vi "ADC.vi"() -> ()   [LabVIEW 2012]
panel:
  out "Current Guess 2":dbl
  out "ADC Output":dbl
  out "Current Guess":dbl
  in  "Slow Conversion?":bool
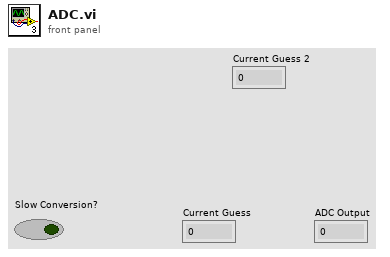
[diagram p1: front panel]
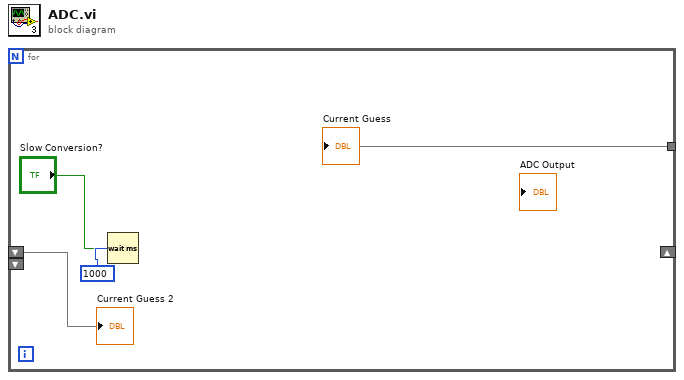
[diagram p0: block diagram]
diagram:
  n1 = for {
    shift-right: _ -> [_]
    shift-left: _ -> [w2]
    shift-left: _ -> [_]
    tunnel: _ -> [w1]
    n2 = Wait (ms)(milliseconds to wait=u32 1000 ("millisecond timer value"), millisecond timer value="Slow Conversion?") -> ()
    "Current Guess" <- w1
    "Current Guess 2" <- w2
  }
